vi "Refresh Status Flags.vi"(8 "error in":errorcluster, 11 "Electronic Load in":refnum<class "Electronic Load.lvclass">) -> (0 "error out":errorcluster, 3 "Electronic Load out":refnum<class "Electronic Load.lvclass">)   [LabVIEW 2019, in "Electronic Load.lvlib" / "Electronic Load.lvclass"]
uses:
  Library/Electronic Load.lvclass
  Library/Electronic Load.lvclass/Electronic Load.ctl
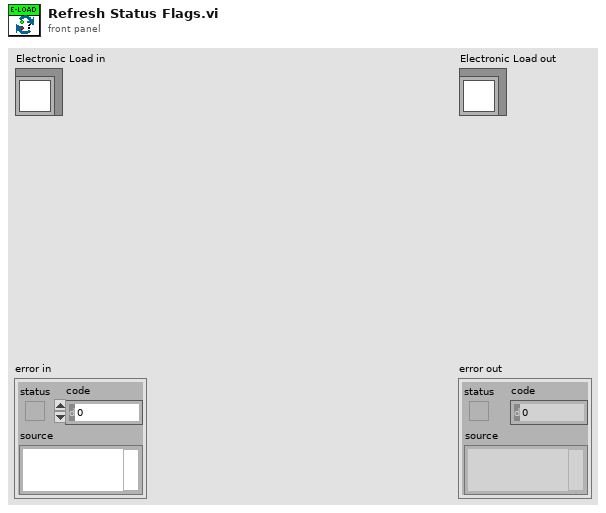
[diagram p1: front panel]
types:
  T1 = typedef "Electronic Load.lvlib/Electronic Load.lvclass/Status_Flags.ctl" = cluster{"Interlock":bool, "OVP":bool, "OCP":bool, "Output":bool}
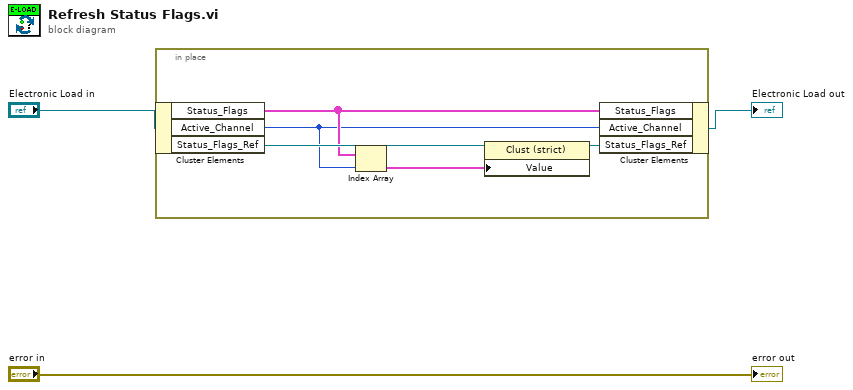
[diagram p0: block diagram]
diagram:
  n1 = in-place {
    n2 = in-place-cluster #1("Electronic Load in") -> ("Status_Flags"=w6:T1[], "Active_Channel"=w5:u32, "Status_Flags_Ref"=w8:refnum<vi>)
    n3 = Index Array(array=w6, index=w5) -> (element=w4:T1)
    n4 = property class="Clust (strict)"(reference=w8, "Value"=w4) -> (reference out=w7:refnum<vi>)  [unwired: 1 in, 1 out]
    n5 = in-place-cluster #1("Status_Flags"=w6, "Active_Channel"=w5, "Status_Flags_Ref"=w7) -> (→"Electronic Load out":refnum<class "Electronic Load.lvclass">)
  }
  "error out" <- "error in"
